vi "LVClass_HasoSlopes Save.vi"(0 "HasoSlopes in":refnum<class "HasoSlopes.lvclass">, 5 "path":path, 7 "comments":string, 9 "session":string, 11 "error in (no error)":errorcluster) -> (4 "HasoSlopes out":refnum<class "HasoSlopes.lvclass">, 15 "error out":errorcluster)   [LabVIEW 2020, in "HasoSlopes.lvclass"]
doc: "Save HasoSlopes to a .has file.\n\n--------------------------------------------------------------------------------\n\n<B>HasoSlopesIn </B> : HasoSlopes object.\n<B>HasoSlopesOut </B> : HasoSlopes object.\n<B>has_file_path </B> : Absolute path to the .has file.\n<B>comments </B> : Comments.\n<B>session_name </B> : Session name.\n<B>ErrorIn </B> : Error\n<B>ErrorOut </B> : Error\n\n--------------------------------------------------------------------------------"
uses:
  HasoSlopes.lvclass
  HasoSlopes.lvclass/HasoSlopes.ctl
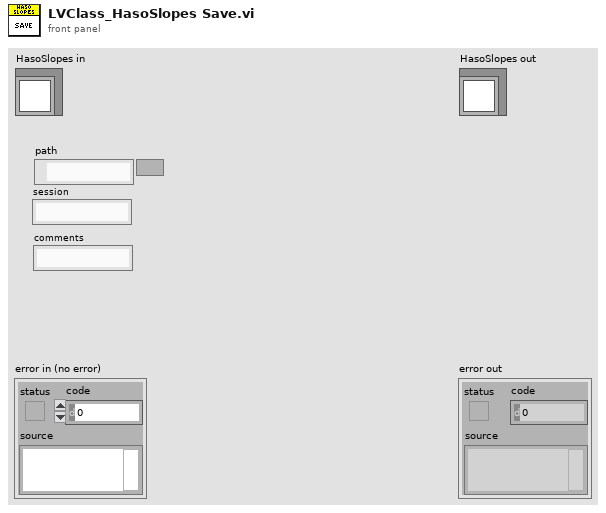
[diagram p1: front panel]
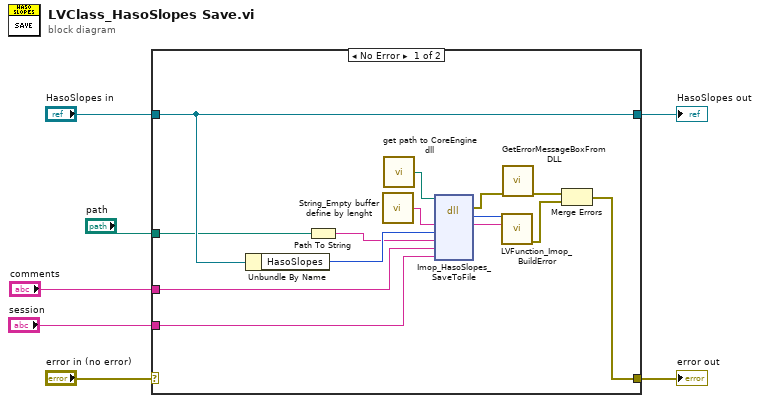
[diagram p0: block diagram]
diagram:
  n1 = case shown="No Error" "error in (no error)" {
    selector: "error in (no error)" -> [_ w23]
    tunnel: [w12 w23] -> w5
    tunnel: [w15 w22] -> w4
    tunnel: "HasoSlopes in" -> [w15 w22]
    tunnel: "path" -> [w10 _]
    tunnel: "comments" -> [w9 _]
    tunnel: "session" -> [w8 _]
    frame No Error {
      n2 = Unbundle By Name(w15) -> ("HasoSlopes"=w16:i32)
      n3 = Path To String(path=w10) -> (string=w11:string)
      n4 = call "String_Empty buffer define by lenght.vi"() -> ("Empty buffer"=w21:string)  [unwired: 1 in]
      n5 = call "get path to CoreEngine dll.vi"() -> ("path to c_interface_vc100.dll"=w18:path)  [unwired: 12 in, 3 out]
      n6 = dll-call lib="D:/soft/HASO_v3/SVN_trunk/ImOpCoreEngine4_LV2011/DLLs/c_interface_vc100.dll" fn="Imop_HasoSlopes_SaveToFile"(path in=w18, "message"=w21, "HasoSlopes"=w16, "Path"=w11, "comments"=w9, "session"=w8) -> (error out=w17:errorcluster, "return type"=w19:i32, "message"=w20:string)  [unwired: 6 in, 1 out]
      n7 = call "LVFunction_Imop_BuildError.vi"("code"=w19, "String to Prepend to source (\"\")"=w20) -> ("error out"=w13:errorcluster)  [unwired: 13 in]
      n8 = call "GetErrorMessageBoxFromDLL.vi"("error IN"=w17) -> ("error OUT"=w14:errorcluster)  [unwired: 10 in]
      n9 = Merge Errors(w14, w13) -> (w12:errorcluster)
    }
    frame Error {
    }
  }
  "error out" <- w5
  "HasoSlopes out" <- w4
